vi "rs3 enable stream.vi"(4 "framerate":u32=30, 6 "format":u16(ring) items=["any", "Depth16", "Disparity16", "f32XYZ", "YUV", "RGB8", "BGR8", "RGBA8", "BGRA8", "Y8", "Y16", "Raw10", "Raw16", "Raw8"], 8 "error in":errorcluster, 9 "size":cluster{"width":u32, "height":u32}, 10 "stream type":u16(ring) items=["depth", "color", "inf 1", "inf 2"], 11 "device":u32) -> (0 "error out":errorcluster, 3 "device":u32)   [LabVIEW 2017, in "libRealSense3.lvlib"]
doc: "Enables the specified stream."
uses:
  <vilib>/addons/RealSense/libRealSense3.lvlib
  <vilib>/addons/RealSense/realsense-d.dll
panel:
  # "RS3 Enable Stream"
  # "(C) Intel Corp.,  AGJ"
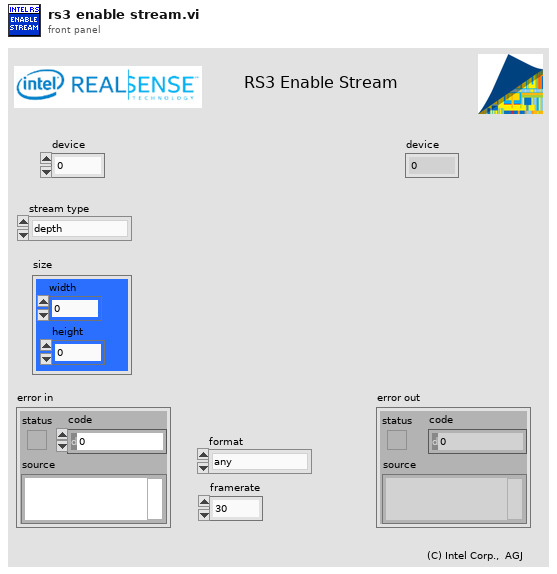
[diagram p1: front panel]
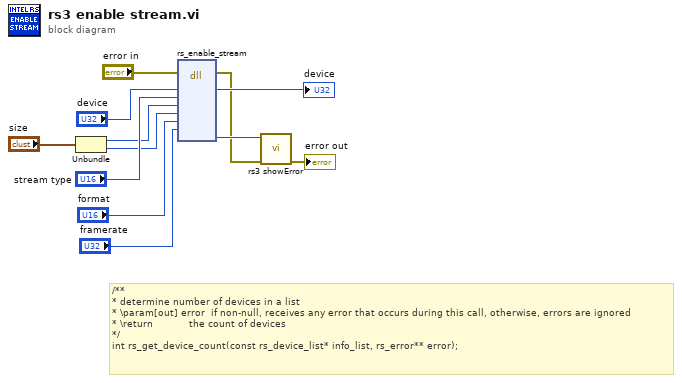
[diagram p0: block diagram]
diagram:
  # "/**\n* determine number of devices in a list\n* \\param[out] error  if non-null, receives any error that occurs during this call, otherwise, errors are ignored\n* \\return            the count of devices\n*/\nint rs_get_device_count(const rs_device_list* info_list, rs_error** error);"
  n1 = Unbundle("size") -> ("width"=w7:u32, "height"=w6:u32)
  n2 = dll-call lib="C:/Program Files (x86)/National Instruments/LabVIEW 2017/vi.lib/addons/RealSense/realsense-d.dll" fn="rs_enable_stream"(error in="error in", "device"="device", "stream_type"="stream type", "width"=w7, "height"=w6, "format"="format", "framerate"="framerate") -> (error out=w2:errorcluster, "device"=→"device":u32, "error"=w3:u64)  [unwired: 9 in, 1 out]
  n3 = call <vilib>:"rs3 showError.vi"("error in (no error)"=w2, "error"=w3) -> ("error out"=→"error out":errorcluster)  [unwired: 5 in, 4 out]
